vi "Core.vi"(8 "error in (no error)":errorcluster, 11 "DemoModule1 in":refnum<class "DemoModule1.lvclass">) -> ()   [LabVIEW 2020, in "Demo.lvlib" / "DemoModule1.lvclass"]
uses:
  DemoModule1.lvclass
  D:/WSGitHub/RTFWK/Realization/Module/Module.lvclass
  <vilib>/Utility/error.llb/Error Cluster From Error Code.vi
  <vilib>/ErrorRing/Error Ring.xnode
  Module/Module.lvclass
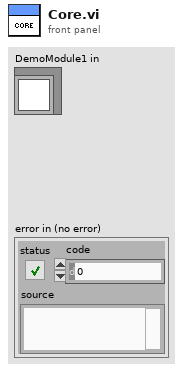
[diagram p1: front panel]
types:
  T1 = enum32{"Invalid", "Standard", "Closed", "Hidden", "Minimized", "Maximized"}
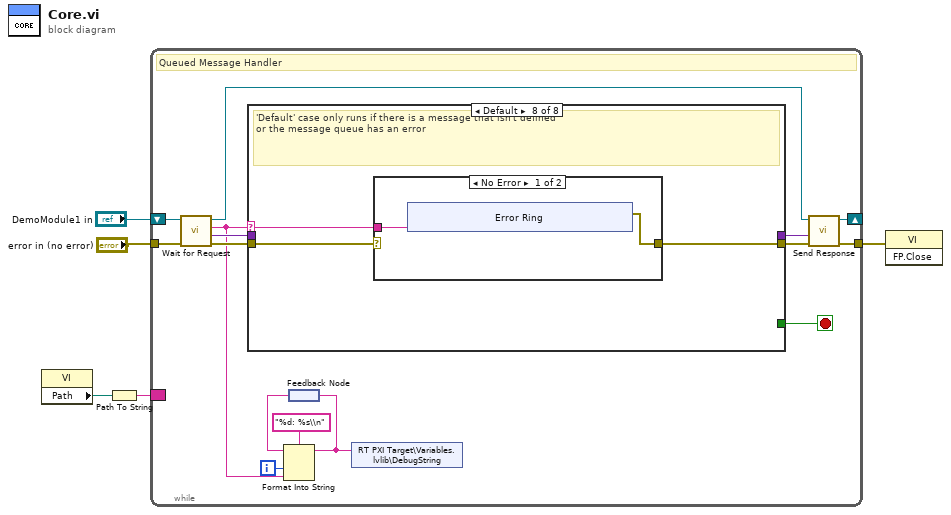
[diagram p0: block diagram]
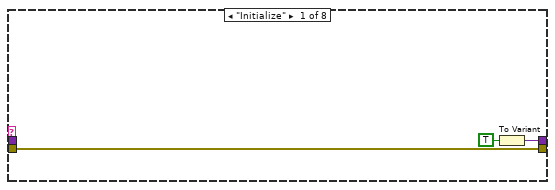
[diagram p2: hidden frame]
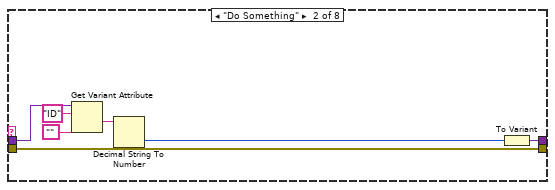
[diagram p3: hidden frame]
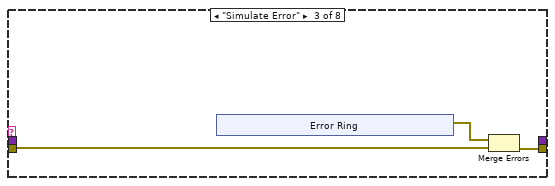
[diagram p4: hidden frame]
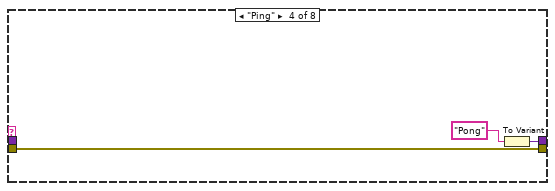
[diagram p5: hidden frame]
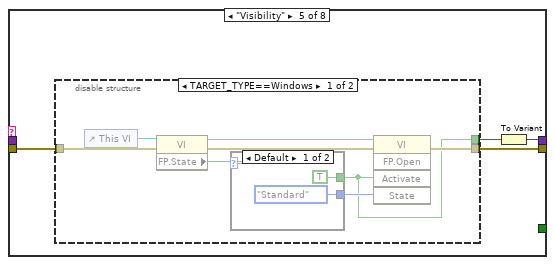
[diagram p6: hidden frame]
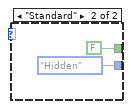
[diagram p7: hidden frame]
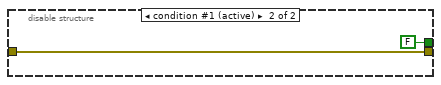
[diagram p8: hidden frame]
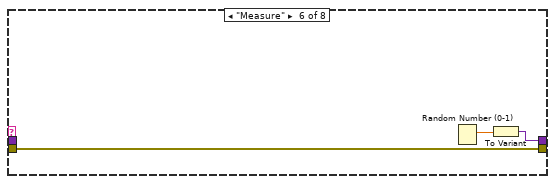
[diagram p9: hidden frame]
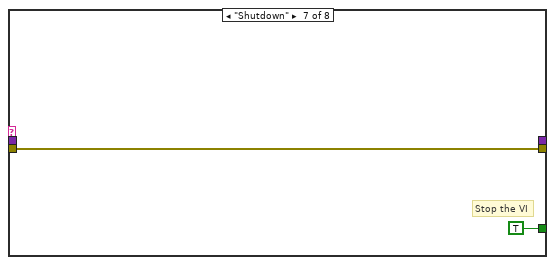
[diagram p10: hidden frame]
diagram:
  n1 = property class="VI"() -> ("Path"=w2:path)  [unwired: 2 in, 2 out]
  n2 = Path To String(path=w2) -> (string=w1:string)
  n3 = while {
    shift-right: [w20] -> _
    shift-left: "DemoModule1 in" -> [w16]
    tunnel: "error in (no error)" -> [w14]
    tunnel: [w17] -> w3
    border: w1 -> [_]
    i -> [w9]
    stop <- w15 stop-if-true
    # "Queued Message Handler"
    n4 = call "Wait for Request.vi"("error in"=w14, "Module in"=w16) -> ("error out"=w13:errorcluster, "Data"=w12:variant, "Message"=w8:string, "Module out"=w11:refnum<class "DemoModule1.lvclass">)  [unwired: 6 in]
    n5 = case shown="Default" w8 {
      selector: w8 -> [_ _ _ _ _ _ _ w66]
      tunnel: w13 -> [w21 w26 w32 w41 w45 w62 w63 w67]
      tunnel: [_ _ _ _ _ _ TRUE _] -> w15
      tunnel: w12 -> [_ w27 _ _ _ _ _ _]
      tunnel: [w23 w25 _ w40 w43 w61 _ _] -> w19
      tunnel: [w21 w26 w33 w41 w44 w62 w63 w65] -> w18
      frame "Initialize" {
        n6 = To Variant(anything=TRUE) -> (Variant=w23:variant)
      }
      frame "Do Something" {
        n7 = Get Variant Attribute(Variant=w27, name="ID", default value (empty Variant)="") -> (value=w28:string)  [unwired: 1 in, 3 out]
        n8 = Decimal String To Number(string=w28) -> (number=w24:i32)  [unwired: 2 in, 1 out]
        n9 = To Variant(anything=w24) -> (Variant=w25:variant)
      }
      frame "Simulate Error" {
        n10 = xnode "Error Ring"() -> ("error out"=w31:errorcluster)
        n11 = Merge Errors(w31, w32) -> (w33:errorcluster)
      }
      frame "Ping" {
        n12 = To Variant(anything="Pong") -> (Variant=w40:variant)
      }
      frame "Visibility" {
        n13 = disable-structure shown="TARGET_TYPE==Windows" {
          disable-tunnel: w45 -> [w53 w59]
          disable-tunnel: [w48 w59] -> w44
          disable-tunnel: [w47 FALSE ("Activate?")] -> w42
          frame condition #0 {
            n14 = control-ref of="This VI"() -> (w46:refnum<vi>)
            n15 = property class="VI"(reference=w46, error in=w53) -> (reference out=w51:refnum<vi>, error out=w52:errorcluster, "FP.State"=w50:T1)
            n16 = case shown="Default" w50 {
              tunnel: [T1."Standard" ("State") T1."Hidden" ("State")] -> w49
              tunnel: [TRUE ("Activate?") FALSE ("Activate?")] -> w47
              frame Default {
              }
              frame "Standard" {
              }
            }
            n17 = invoke class="VI" method="FP.Open"(reference=w51, error in=w52, "Activate"=w47, "State"=w49) -> (error out=w48:errorcluster)  [unwired: 1 in, 4 out]
          }
          frame condition #1 (active) {
          }
        }
        n18 = To Variant(anything=w42) -> (Variant=w43:variant)
      }
      frame "Measure" {
        n19 = Random Number (0-1)() -> (number: 0 to 1=w60:dbl)
        n20 = To Variant(anything=w60) -> (Variant=w61:variant)
      }
      frame "Shutdown" {
        # "Stop the VI"
      }
      frame Default {
        # "'Default' case only runs if there is a message that isn't defined\nor the message queue has an error"
        n21 = case shown="No Error" w67 {
          selector: w67 -> [_ w77]
          tunnel: w66 -> [w69 _]
          tunnel: [w68 w77] -> w65
          frame No Error {
            n22 = xnode ("Error Ring")("parameter 0"=w69) -> ("error out"=w68:errorcluster)
          }
          frame Error {
          }
        }
      }
    }
    n23 = feedback #1() -> (w7:string)
    n24 = Format Into String(format string="%d: %s\\n", initial string=w7, w9, w8) -> (resulting string=w6:string)  [unwired: 1 in, 1 out]
    n25 = feedback-in #1(w6) -> ()
    n26 = shared-variable "RT PXI Target\\Variables.lvlib\\DebugString"(w6) -> ()  [unwired: 1 in, 1 out]
    n27 = call "Send Response.vi"("error in"=w18, "Response"=w19, "Module in"=w11) -> ("error out"=w17:errorcluster, "Module out"=w20:refnum<class "DemoModule1.lvclass">)  [unwired: 7 in]
  }
  n28 = invoke class="VI" method="FP.Close"(error in=w3) -> ()  [unwired: 2 in, 3 out]
